vi "Page_Info_Initialize.vi"(8 "error in (no error)":errorcluster, 9 "ctlReferences":T1, 10 "Target file visible? (T)":bool=TRUE, 11 "Build in":refnum<class "AB_Build.lvclass">) -> (0 "error out":errorcluster, 3 "Build out":refnum<class "AB_Build.lvclass">)   [LabVIEW 2020, in "AB_Deployment.lvlib"]
uses:
  <vilib>/AppBuilder/AB_Classes/Deployment/AB_Deployment.lvlib
  <vilib>/AppBuilder/AB_Classes/Build/AB_Build.lvclass
  <resource>/Framework/Providers/Builds/AppBuilder/AB_UI_Page_Info_References.ctl
  <resource>/Framework/Providers/Common/provcom_StringGlobals.vi
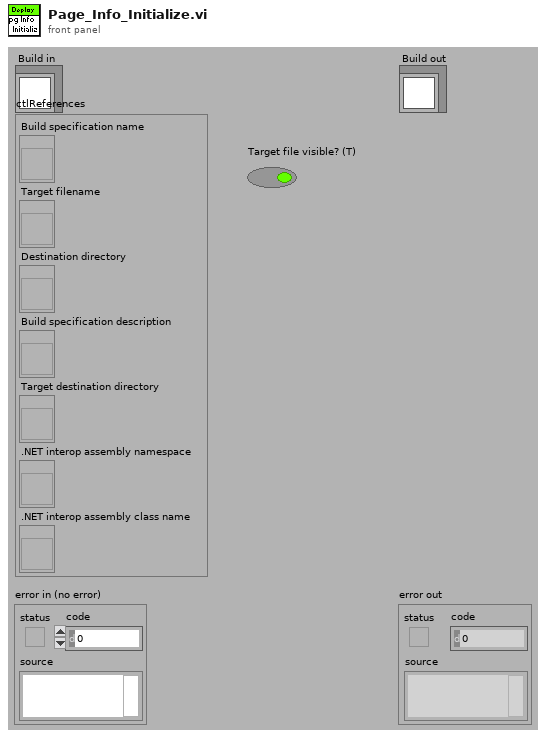
[diagram p1: front panel]
types:
  T1 = typedef "AB_UI_Page_Info_References.ctl" = cluster{"Build specification name":refnum<vi>, "Target filename":refnum<vi>, "Destination directory":refnum<vi>, "Build specification description":refnum<vi>, "Target destination directory":refnum<vi>, ".NET interop assembly namespace":refnum<vi>, ".NET interop assembly class name":refnum<vi>}
  T2 = typedef "LVRectTypeDef.ctl" = cluster{"Left":i16, "Top":i16, "Right":i16, "Bottom":i16}
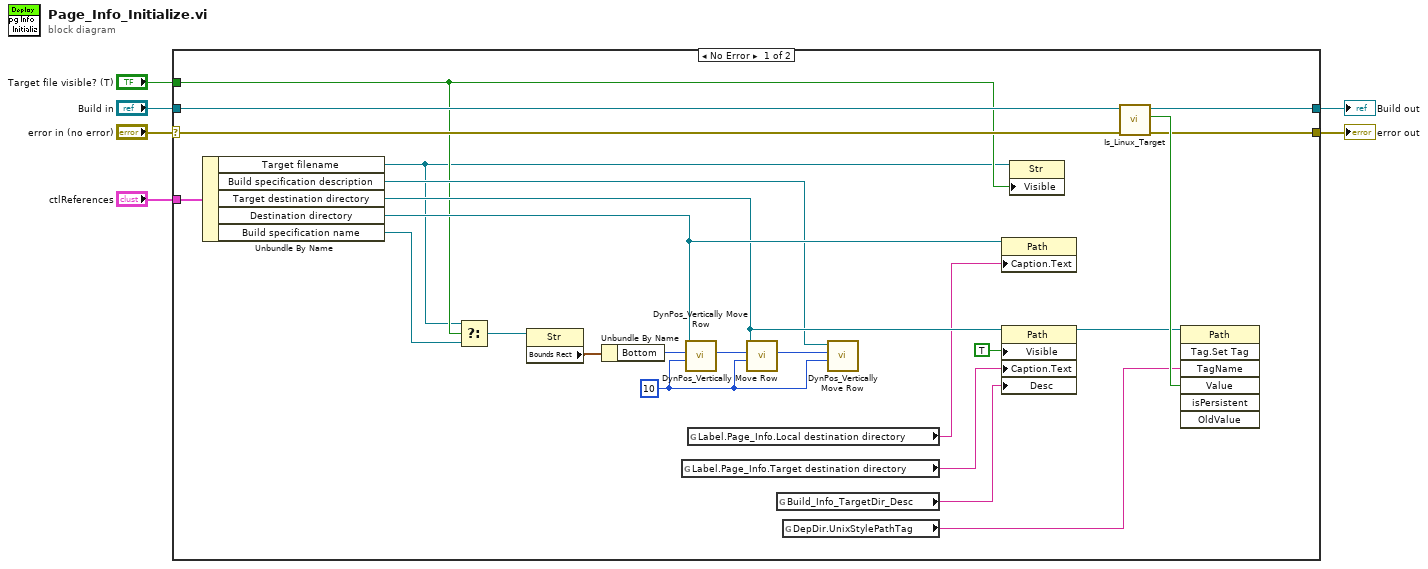
[diagram p0: block diagram]
diagram:
  n1 = case shown="No Error" "error in (no error)" {
    selector: "error in (no error)" -> [w14 w32]
    tunnel: [w13 w32] -> w5
    tunnel: [w15 w31] -> w2
    tunnel: "Build in" -> [w16 w31]
    tunnel: "ctlReferences" -> [w28 _]
    tunnel: "Target file visible? (T)" -> [w9 _]
    frame No Error {
      w21 = 10 ("Pixel separation (6)")
      n2 = Unbundle By Name(w28) -> ("Target filename"=w8:refnum<vi>, "Build specification description"=w23:refnum<vi>, "Target destination directory"=w24:refnum<vi>, "Destination directory"=w25:refnum<vi>, "Build specification name"=w10:refnum<vi>)
      n3 = Select(t=w8, s=w9, f=w10) -> (s? t:f=w7:refnum<vi>)
      n4 = property class="Str"(reference=w7) -> ("Bounds Rect"=w30:T2)  [unwired: 1 in, 2 out]
      n5 = Unbundle By Name(w30) -> ("Bottom"=w29:i16)
      n6 = global read "provcom_StringGlobals.vi" "Label.Page_Info.Target destination directory"() -> (w19:string)
      n7 = call <vilib>:"DynPos_Vertically Move Row.vi"("Pixel separation (6)"=w21, "Bottom of last control"=w29, "Control"=w25) -> ("Bottom pixel"=w27:i32)  [unwired: 1 in, 7 out]
      n8 = global read "provcom_StringGlobals.vi" "Label.Page_Info.Local destination directory"() -> (w20:string)
      n9 = call <vilib>:"DynPos_Vertically Move Row.vi"("Pixel separation (6)"=w21, "Bottom of last control"=w27, "Control"=w24) -> ("Bottom pixel"=w22:i32)  [unwired: 1 in, 7 out]
      n10 = global read "provcom_StringGlobals.vi" "Build_Info_TargetDir_Desc"() -> (w18:string)
      n11 = global read "provcom_StringGlobals.vi" "DepDir.UnixStylePathTag"() -> (w11:string)
      n12 = call <vilib>:"DynPos_Vertically Move Row.vi"("Pixel separation (6)"=w21, "Bottom of last control"=w22, "Control"=w23) -> ()  [unwired: 1 in, 8 out]
      n13 = property class="Path"(reference=w25, "Caption.Text"=w20) -> ()  [unwired: 1 in, 2 out]
      n14 = property class="Path"(reference=w24, "Visible"=TRUE, "Caption.Text"=w19, "Desc"=w18) -> (reference out=w12:refnum<vi>)  [unwired: 1 in, 1 out]
      n15 = property class="Str"(reference=w8, "Visible"=w9) -> ()  [unwired: 1 in, 2 out]
      n16 = call <vilib>:"Is_Linux_Target.vi"("error in (no error)"=w14, "AB_Build in"=w16) -> ("error out"=w13:errorcluster, "Linux?"=w17:bool, "AB_Build out"=w15:refnum<class "AB_Build.lvclass">)  [unwired: 7 in]
      n17 = invoke class="Path" method="Tag.Set Tag"(reference=w12, "TagName"=w11, "Value"=w17) -> ()  [unwired: 4 in, 7 out]
    }
    frame Error {
    }
  }
  "error out" <- w5
  "Build out" <- w2
